vi "BVR Probe.vi"(11 "ByRef Variant Repsitory out":refnum<data-value>) -> (2 "Value String":string, 3 "Boolean":bool)   [LabVIEW 2015]
panel:
  in  "Type":enum16{""}(ring)
  in  "Tag":string
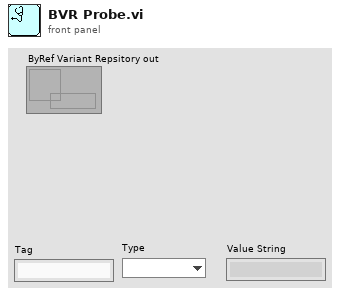
[diagram p1: front panel]
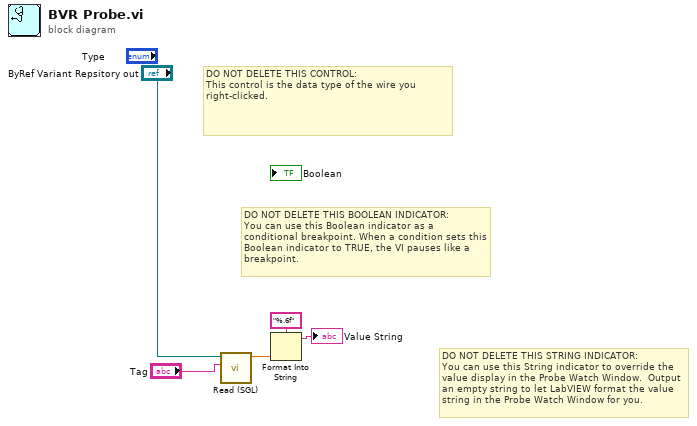
[diagram p0: block diagram]
diagram:
  # "DO NOT DELETE THIS STRING INDICATOR: \nYou can use this String indicator to override the value display in the Probe Watch Window.  Output an empty string to let LabVIEW format the value string in the Probe Watch Window for you."
  # "DO NOT DELETE THIS BOOLEAN INDICATOR: \nYou can use this Boolean indicator as a conditional breakpoint. When a condition sets this Boolean indicator to TRUE, the VI pauses like a breakpoint."
  # "DO NOT DELETE THIS CONTROL: \nThis control is the data type of the wire you right-clicked."
  n1 = call "Read (SGL).vi"("Tag"="Tag", "ByRef Variant Repsitory in"="ByRef Variant Repsitory out") -> ("Value"=w2:sgl)  [unwired: 7 in, 1 out]
  n2 = Format Into String(format string="%.6f", w2) -> (resulting string=→"Value String":string)  [unwired: 2 in, 1 out]
